vi "Process Ch2v2.vi"(11 "Init?":bool) -> (2 "Max1":u32, 3 "Max0":u32)   [LabVIEW 2018]
uses:
  <vilib>/rvi/Emulation/niFpgaGetClockAttributes.vi
  <vilib>/rvi/Emulation/niFpgaSctlEmulationGetInTimedLoop.vi
  <vilib>/rvi/Emulation/niFpgaEmulationReportErrorSimple.vi
  <vilib>/rvi/Emulation/niFpgaEmulationIsFPGAContextNoSignature.vi
  <vilib>/rvi/DataTransferAndStorage/Container/Common/niFpgaContainerGetUniqueNameForEmu.vi
  <vilib>/rvi/Memory/Memory_Emulation/niFpgaMemoryEmulationCacheClearOnFirstRun.vi
  <vilib>/rvi/Memory/Memory_Emulation/nirvimemoryEmulationManagerCache_MakeExclusive.vi
  <vilib>/rvi/Memory/Memory_Emulation/niFpgaMemoryEmulationValidateCache.vi
  <vilib>/rvi/Memory/Memory_Emulation/nirvimemoryEmulationManagerCache_InsertValue.vi
  <vilib>/Utility/error.llb/Clear Errors.vi
  <vilib>/rvi/Memory/Memory_Emulation/nirvimemoryEmulationManagerCache_ReleaseExclusive.vi
  <vilib>/rvi/Memory/Memory_Emulation/nirvimemoryEmulationManagerCache_GetValue.vi
  <vilib>/rvi/Memory/Memory_Emulation/nirvimemoryEmulationManagerCache_SetValue.vi
  <vilib>/rvi/Emulation/niFpgaProcessEmulError.vi
  <vilib>/rvi/FIFO/Fifo_Resource/nirvififoEmulationSetSize.vi
  <vilib>/rvi/FIFO/Fifo_Resource/nirviFifoEmulationQueueMgr.vi
  <instcachedir>/0/nirviFifoEmulationQueueMgr_E5CAEC123FF24DC58D834DCA3CDAA9B5.lvgen/nirviFifoEmulationQueueMgr_E5CAEC123FF24DC58D834DCA3CDAA9B5_001.vi
  <vilib>/rvi/Memory/Memory_Emulation/nirvimemoryFastEmulation.vi
  <vilib>/rvi/Memory/Memory_Emulation/nirvimemoryEmulation.vi
  <vilib>/rvi/errors/nirviReportUnexpectedCaseInternalError (U32).vi
  <vilib>/rvi/DataTransferAndStorage/Container/Common/niFpgaContainerExecOnDevCompGetState.vi
  <vilib>/rvi/Emulation/niFpgaSctlEmulationResourceMgr.vi
  <vilib>/rvi/errors/niFpgaSetErrorForExecOnDevCompSimple.vi
  <vilib>/rvi/eio/common/nirviEmuReportErrorAndStop.vi
  <vilib>/rvi/FIFO/Fifo_Resource/nirvififoEmulationCreateLock.vi
  <vilib>/rvi/FIFO/Fifo_Resource/nirvififoEmulationObtainLock.vi
  <vilib>/rvi/FIFO/Fifo_Resource/nirvififoEmulationReleaseLock.vi
  <vilib>/rvi/occurrence/nirviWaitOnOccurrenceBase.vi
  <vilib>/rvi/errors/nirviReportUnexpectedCaseInternalError.vi
  <vilib>/rvi/Emulation/niFpgaCriticalErrorInLSC.vi
  <vilib>/rvi/DataTransferAndStorage/Container/XNode/niFpgaContainer.xnode
  <vilib>/rvi/DataTransferAndStorage/Register/Emulation/niFpgaRegisterEmulation.vi
  <vilib>/rvi/FIFO/Fifo_Resource/nirvififoEmulationGetNumberOfElementsToRead.vi
  <vilib>/rvi/Memory/Memory_Emulation/niFpgaMemoryEmulationRefIn.vi
  <vilib>/rvi/FIFO/Fifo_Resource/nirvififoEmulationRead.vi
  <vilib>/rvi/FXPMathLib/FxpSub/XNode/nifxpmath_Sub.xnode
  <vilib>/rvi/FXPMathLib/sim/FxpSim.dll
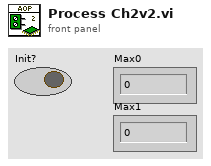
[diagram p1: front panel]
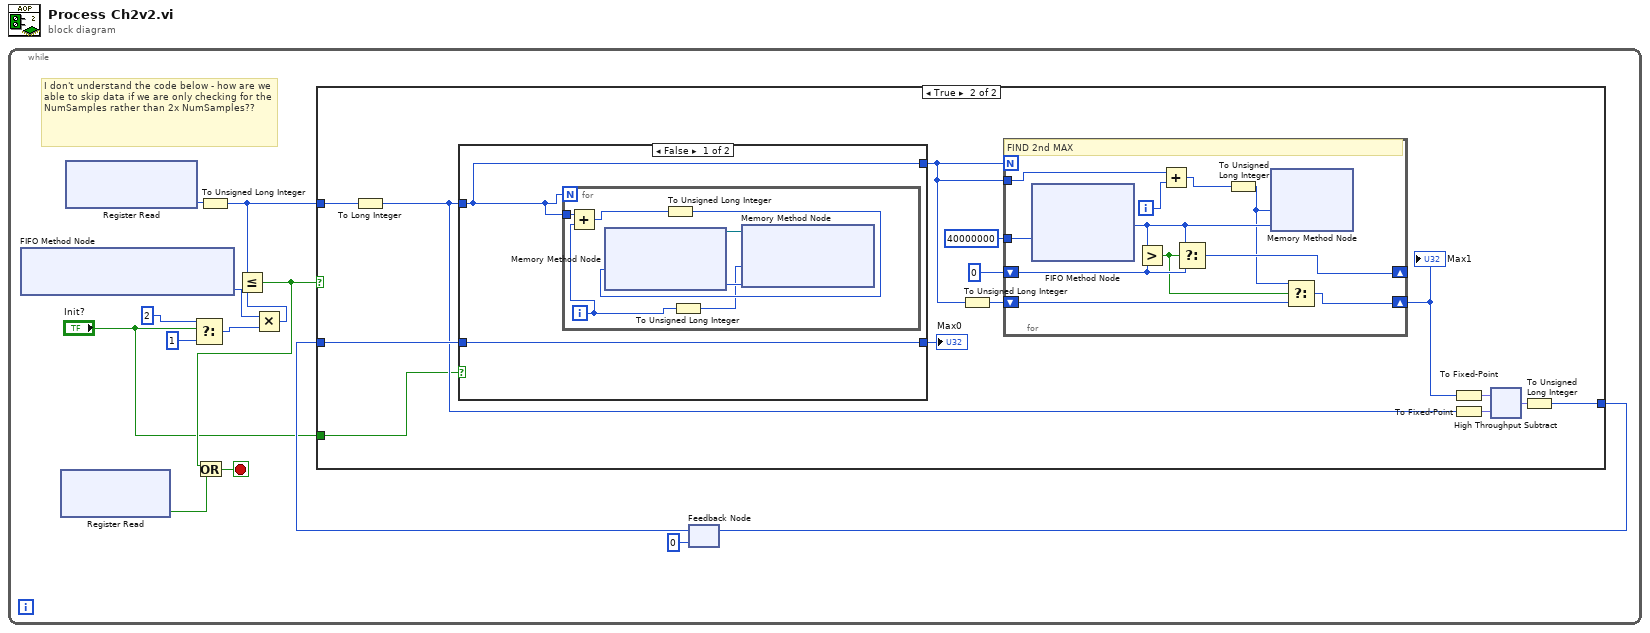
[diagram p0: block diagram]
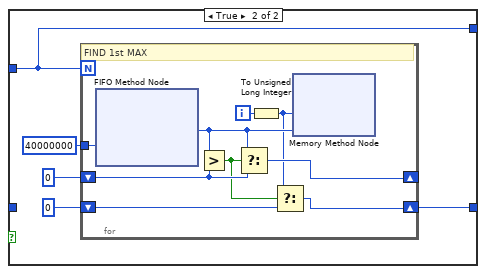
[diagram p3: hidden frame]
diagram:
  n1 = while {
    stop <- w11 stop-if-true
    # "I don't understand the code below - how are we able to skip data if we are only checking for the NumSamples rather than 2x NumSamples??"
    n2 = xnode ("FIFO Method Node")() -> ("Number of Elements to Read"=w7:u32)  [unwired: 1 in, 1 out]
    n3 = xnode ("Register Read")() -> ("Data"=w12:bool)  [unwired: 1 in, 1 out]
    n4 = xnode ("Register Read")() -> ("Data"=w9:u16)  [unwired: 1 in, 1 out]
    n5 = Select(t=u32 2 ("Number of Elements to Read"), s="Init?", f=u32 1) -> (s? t:f=w6:u32)
    n6 = To Unsigned Long Integer(number=w9) -> (unsigned 32bit integer=w8:u32)
    n7 = Multiply(x=w7, y=w6) -> (x*y=w3:u32)
    n8 = Less Or Equal?(x=w8, y=w3) -> (x <= y?=w2:bool)
    n9 = Or(x=w2, y=w12) -> (x .or. y?=w11:bool)
    n10 = feedback #1(u32 0) -> (w14:u32)
    n11 = case shown="True" w2 {
      tunnel: w8 -> [_ w29]
      tunnel: w14 -> [w15 w28]
      tunnel: [w15 w27] -> w10
      tunnel: "Init?" -> [_ w19]
      frame False {
      }
      frame True {
        n12 = To Long Integer(number=w29) -> (32bit integer=w22:i32)
        n13 = case shown="False" w19 {
          tunnel: [w31 w43] -> w21
          tunnel: w22 -> [w30 w39]
          tunnel: w28 -> [w31 _]
          tunnel: [w30 w39] -> w20
          frame False {
            n14 = for {
              N: w30 -> [_]
              tunnel: w30 -> [w38]
              i -> [w33]
              n15 = Add(x=w38, y=w33) -> (x+y=w35:i32)
              n16 = To Unsigned Long Integer(number=w35) -> (unsigned 32bit integer=w34:u32)
              n17 = xnode ("Memory Method Node")("Address"=w34) -> ("Data"=w36:i16, "Memory Out"=w37:refnum<k21>)  [unwired: 1 in]
              n18 = To Unsigned Long Integer(number=w33) -> (unsigned 32bit integer=w32:u32)
              n19 = xnode ("Memory Method Node")("Address"=w32, "Data"=w36, "Memory In"=w37) -> ()  [unwired: 1 out]
            }
          }
          frame True {
            n20 = for {
              N: w39 -> [_]
              shift-right: [w50] -> _
              shift-left: i16 0 ("Element") -> [w51]
              shift-right: [w47] -> w43
              shift-left: u32 0 ("Element") -> [w48]
              tunnel: 40000000 ("Timeout") -> [w44]
              i -> [w46]
              # "FIND 1st MAX"
              n21 = xnode ("FIFO Method Node")("Timeout"=w44) -> ("Element"=w52:i16)  [unwired: 1 in, 2 out]
              n22 = Greater?(x=w52, y=w51) -> (0:w49:bool)
              n23 = Select(t=w52, s=w49, f=w51) -> (s? t:f=w50:i16)
              n24 = To Unsigned Long Integer(number=w46) -> (unsigned 32bit integer=w45:u32)
              n25 = Select(t=w45, s=w49, f=w48) -> (s? t:f=w47:u32)
              n26 = xnode ("Memory Method Node")("Address"=w45, "Data"=w52) -> ()  [unwired: 1 in, 1 out]
            }
          }
        }
        "Max0" <- w21
        n27 = To Unsigned Long Integer(number=w20) -> (unsigned 32bit integer=w25:u32)
        n28 = for {
          N: w20 -> [_]
          shift-right: [w61] -> _
          shift-left: i16 0 ("Element") -> [w62]
          shift-right: [w58] -> w24
          shift-left: w25 -> [w59]
          tunnel: 40000000 ("Timeout") -> [w56]
          tunnel: w20 -> [w54]
          i -> [w55]
          # "FIND 2nd MAX"
          n29 = xnode ("FIFO Method Node")("Timeout"=w56) -> ("Element"=w63:i16)  [unwired: 1 in, 2 out]
          n30 = Greater?(x=w63, y=w62) -> (0:w60:bool)
          n31 = Add(x=w54, y=w55) -> (x+y=w53:i32)
          n32 = Select(t=w63, s=w60, f=w62) -> (s? t:f=w61:i16)
          n33 = To Unsigned Long Integer(number=w53) -> (unsigned 32bit integer=w57:u32)
          n34 = xnode ("Memory Method Node")("Address"=w57, "Data"=w63) -> ()  [unwired: 1 in, 1 out]
          n35 = Select(t=w57, s=w60, f=w59) -> (s? t:f=w58:u32)
        }
        "Max1" <- w24
        n36 = To Fixed-Point(number=w24) -> (fixed-point=w18:fxp<+,32,32>)  [unwired: 1 in]
        n37 = To Fixed-Point(number=w22) -> (fixed-point=w16:fxp<+/-,32,32>)  [unwired: 1 in]
        n38 = xnode "High Throughput Subtract"("x"=w18, "y"=w16) -> ("x-y"=w17:fxp<+,32,32>)
        n39 = To Unsigned Long Integer(number=w17) -> (unsigned 32bit integer=w27:u32)
      }
    }
    n40 = feedback-in #1(w10) -> ()
  }
